vi "setMagnet.vi"(4 "Mode":T2, 6 "Axis":T1=enum."Z", 8 "error in (no error)":errorcluster, 9 "Target Rate (T/min)":dbl, 10 "Target Field (T)":dbl, 11 "Instrument.Oxford1820 in":refnum<class "Instrument.Oxford1820.lvclass">) -> (0 "error out":errorcluster, 3 "Instrument.Oxford1820 out":refnum<class "Instrument.Oxford1820.lvclass">)   [LabVIEW 2019, in "Instrument.Oxford1820.lvclass"]
uses:
  Instrument.Oxford1820.lvclass
  <userlib>/LevyLab/Instrument Framework/Instrument Types/Cryostat/Instrument.Cryostat.lvclass
  <userlib>/LevyLab/Instrument Framework/Instrument Types/Cryostat/Typedefs/Magnet Mode--Enum.ctl
  <userlib>/LevyLab/Instrument Framework/Instrument Types/Cryostat/Typedefs/Magnet Axis--Enum.ctl
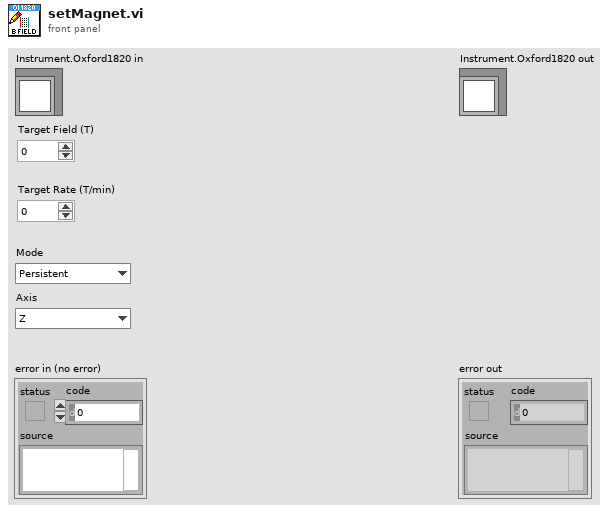
[diagram p1: front panel]
types:
  T1 = typedef "Instrument.Cryostat.lvclass/Magnet Axis--Enum.ctl" = enum16{"X", "Y", "Z"}
  T2 = typedef "Instrument.Cryostat.lvclass/Magnet Mode--Enum.ctl" = enum16{"Persistent", "Driven"}
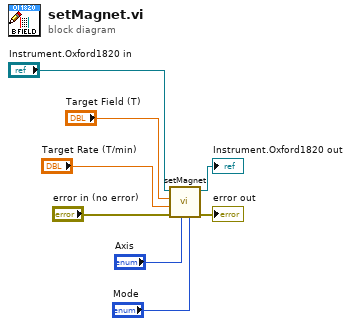
[diagram p0: block diagram]
diagram:
  n1 = call-parent "setMagnet.vi"("Mode"="Mode", "Axis"="Axis", "error in (no error)"="error in (no error)", "Target Rate (T/min)"="Target Rate (T/min)", "Target Field (T)"="Target Field (T)", "Instrument.Cryostat in"="Instrument.Oxford1820 in") -> ("error out"=→"error out":errorcluster, "Instrument.Cryostat out"=→"Instrument.Oxford1820 out":refnum<class "Instrument.Oxford1820.lvclass">)  [unwired: 4 in]
